vi "CaseStructure.vi"() -> ()   [LabVIEW 2018]
panel:
  in  "Boolean":bool
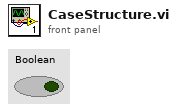
[diagram p1: front panel]
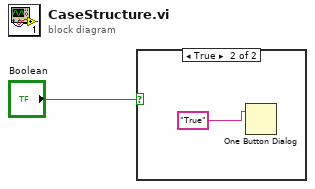
[diagram p0: block diagram]
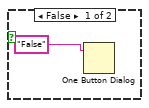
[diagram p2: hidden frame]
diagram:
  n1 = case shown="True" "Boolean" {
    frame False {
      n2 = One Button Dialog(message="False") -> ()  [unwired: 1 in, 1 out]
    }
    frame True {
      n3 = One Button Dialog(message="True") -> ()  [unwired: 1 in, 1 out]
    }
  }
